vi "donut Animate.vi"() -> ()   [LabVIEW 2011]
doc: "This VI demonstrates how to animate a picture on the front panel using a picture ring (Pict Ring) control. This VI takes a sequence of pictures where each picture represents a \"frame\" of the animaction and makes each picture a selection in the picture ring. By programmatically incrementing the value of the picture ring, the picture appears to be animated."
panel:
  in  "停止":bool
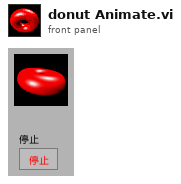
[diagram p1: front panel]
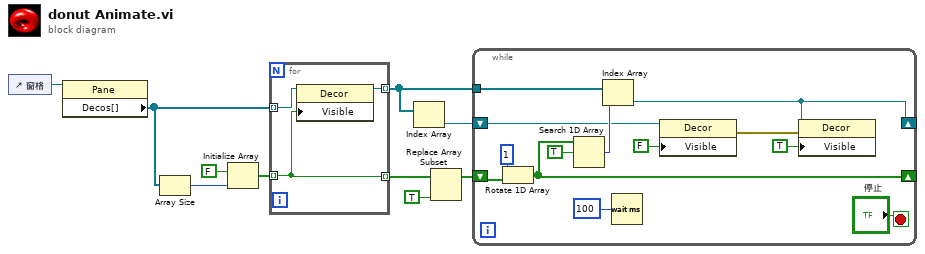
[diagram p0: block diagram]
diagram:
  n1 = control-ref of="窗格"() -> (w10:refnum<vi>)
  n2 = property class="Pane"(reference=w10) -> ("Decos[]"=w5:refnum<vi>[])  [unwired: 1 in, 2 out]
  n3 = Array Size(array=w5) -> (size(s)=w9:i32)
  n4 = Initialize Array(FALSE, w9) -> (w4:bool[])
  n5 = for {
    tunnel: w5 -> [w13] mode=indexing
    tunnel: w4 -> [w12] mode=indexing
    tunnel: [w12] -> w3 mode=indexing
    tunnel: [w11] -> w1 mode=indexing
    n6 = property class="Decor"(reference=w13, "Visible"=w12) -> (reference out=w11:refnum<vi>)  [unwired: 1 in, 1 out]
  }
  n7 = Index Array(array=w1) -> (element=w2:refnum<vi>)  [unwired: 1 in]
  n8 = Replace Array Subset(array=w3, new element=TRUE ("新元素/子数组")) -> (w6:bool[])  [unwired: 1 in]
  n9 = while {
    shift-right: [w16] -> _
    shift-left: w6 -> [w23]
    tunnel: w1 -> [w19]
    shift-right: [w15] -> _
    shift-left: w2 -> [w14]
    stop <- "停止" stop-if-true
    n10 = Rotate 1D Array(1:w23, 2:1 ("n")) -> (0:w16:bool[])
    n11 = Search 1D Array(1D array=w16, element=TRUE ("元素")) -> (index of element=w20:i32)  [unwired: 1 in]
    n12 = Index Array(array=w19, index=w20) -> (element=w15:refnum<vi>)
    n13 = Wait (ms)(milliseconds to wait=u32 100 ("等待时间（毫秒）")) -> ()  [unwired: 1 out]
    n14 = property class="Decor"(reference=w14, "Visible"=FALSE ("可见")) -> (error out=w17:errorcluster)  [unwired: 1 in, 1 out]
    n15 = property class="Decor"(reference=w15, error in=w17, "Visible"=TRUE ("可见")) -> ()  [unwired: 2 out]
  }
